vi "CaculateCheckSum.vi"(11 "hex":string="\bU\u0004\u0000\u0000\u0000\u0001\u0000b") -> (3 "hex include checksum":string)   [LabVIEW 2018]
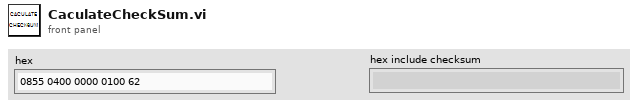
[diagram p1: front panel]
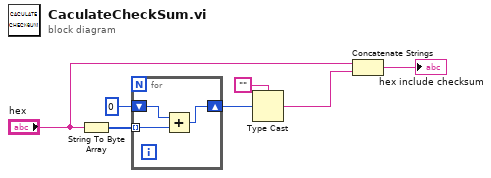
[diagram p0: block diagram]
diagram:
  n1 = String To Byte Array(string="hex") -> (unsigned byte array=w7:u8[])
  n2 = for {
    tunnel: w7 -> [w10] mode=indexing
    shift-right: [w8] -> w3
    shift-left: u8 0 -> [w9]
    n3 = Add(x=w9, y=w10) -> (x+y=w8:u8)
  }
  n4 = Type Cast(type="", x=w3) -> (*(type *) &x=w1:string)
  n5 = Concatenate Strings("hex", w1) -> (→"hex include checksum":string)
